vi "FormatBoolean.vi"(1 "value":bool) -> (0 "python object":string)   [LabVIEW 2014, in "Python Functions.lvlib"]
uses:
  Python Functions.lvlib
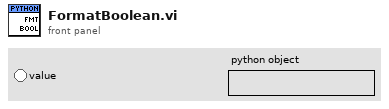
[diagram p1: front panel]
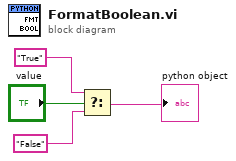
[diagram p0: block diagram]
diagram:
  n1 = Select(t="True", s="value", f="False") -> (s? t:f=→"python object":string)
